vi "Momentum_Killer_2017_loop.vi"() -> ()   [LabVIEW 2016]
panel:
  out "Power Output":dbl
  in  "Power Input":dbl
  in  "Kill Control":bool
  in  "Stop Delay (sec)":dbl=0.5
  in  "Reverse Time (sec)":dbl
  in  "Edge":bool
  in  "Reverse Power":dbl
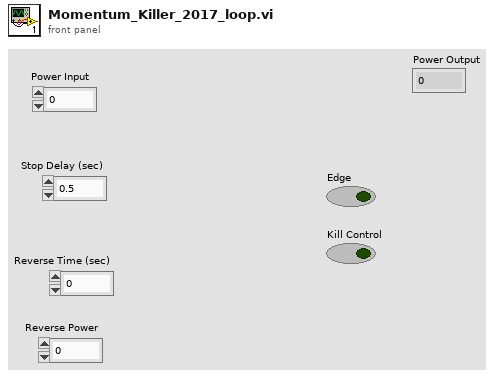
[diagram p1: front panel]
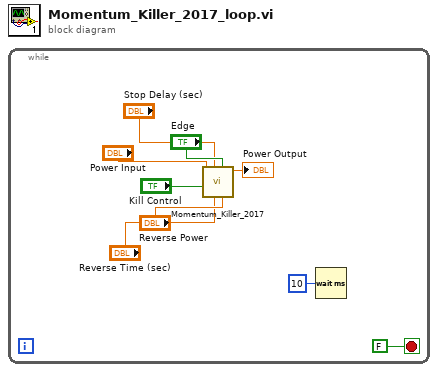
[diagram p0: block diagram]
diagram:
  n1 = while {
    stop <- FALSE stop-if-true
    n2 = call <userlib>:"Momentum_Killer_2017.vi"("Reverse Power"="Reverse Power", "Edge"="Edge", "Reverse Time (sec)"="Reverse Time (sec)", "Stop Delay (sec)"="Stop Delay (sec)", "Kill Control"="Kill Control", "Power Input"="Power Input") -> ("Power Output"=→"Power Output":dbl)  [unwired: 5 in]
    n3 = Wait (ms)(milliseconds to wait=u32 10) -> ()  [unwired: 1 out]
  }
